vi "Load Config.vi"(8 "error in (no error)":errorcluster, 11 "SoftVar Module in":refnum<class "SoftVar Module.lvclass">) -> (0 "error out":errorcluster, 3 "SoftVar Module out":refnum<class "SoftVar Module.lvclass">)   [LabVIEW 2020, in "Volatus.lvlib" / "SoftVar Module.lvclass"]
uses:
  SoftVar Module.lvclass
  C:/dev/lv20CE/relink/lv-volatus/Volatus/Module/Module.lvclass
  Module/Module.lvclass/Module.ctl
  VolatusConfig/VolatusConfigElement/VolatusConfigElement.lvclass/VolatusConfigElement.ctl
  SoftVar Module.lvclass/SoftVar Module.ctl
  lv-vecto/Vecto/Group/Group.lvclass
  C:/dev/lv20CE/relink/lv-vecto/Vecto/GroupAbstract/GroupAbstract.lvclass
  Module/Config.vi
  VolatusConfig/VolatusConfigElement/Element.vi
  VolatusConfig/Task/Task.lvclass
  C:/dev/lv20CE/relink/lv-volatus/VolatusConfig/VolatusConfigElement/VolatusConfigElement.lvclass
  Module/Module.lvclass
  VolatusConfig/VolatusConfigElement/VolatusConfigElement.lvclass
  lv-cdm/CDM-Config/Config Element/Config Element.lvclass
  C:/dev/lv20CE/relink/lv-volatus/Volatus/SoftVar Module/SoftVar Module.lvclass
  VolatusConfig/Group/Group.lvclass
  VolatusConfig/Endpoint.ctl
  VolatusConfig/VolatusConfig.lvlib
  C:/dev/lv20CE/relink/lv-volatus/VolatusConfig/Task/Task.lvclass
  C:/dev/lv20CE/relink/lv-vecto/Vecto/Group/Group.lvclass
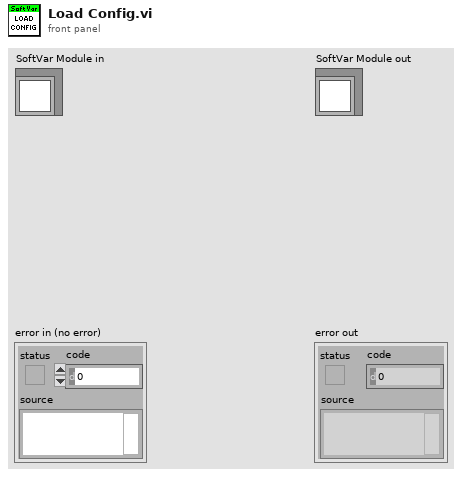
[diagram p1: front panel]
types:
  T1 = typedef "VolatusConfig.lvlib/Endpoint.ctl" = cluster{"Address":string, "Port":u16}
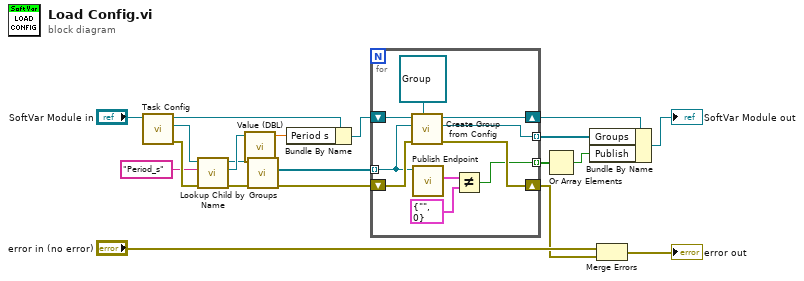
[diagram p0: block diagram]
diagram:
  n1 = call "Task Config.vi"("Module in"="SoftVar Module in") -> ("error out"=w20:errorcluster, "Task Config"=w16:refnum<class "Task.lvclass">, "Module out"=w17:refnum<class "SoftVar Module.lvclass">)  [unwired: 8 in]
  n2 = call "Lookup Child by Name.vi"("error in (no error)"=w20, "Child Name"="Period_s", "VolatusConfigElement in"=w16) -> ("error out"=w11:errorcluster, "Child"=w14:refnum<class "Config Element.lvclass">, "VolatusConfigElement out"=w12:refnum<class "Task.lvclass">)  [unwired: 5 in, 1 out]
  n3 = call "Value (DBL).vi"("Config Element in"=w14) -> ("DBL Value"=w13:dbl)  [unwired: 9 in, 1 out]
  n4 = call "Groups.vi"("error in (no error)"=w11, "Task in"=w12) -> ("error out"=w7:errorcluster, "Groups"=w8:refnum<class "Group.lvclass">[])  [unwired: 7 in, 1 out]
  n5 = Bundle By Name(cluster=w17, "Period s"=w13) -> (w10:refnum<class "SoftVar Module.lvclass">)
  n6 = for {
    shift-right: [w26] -> w9
    shift-left: w10 -> [w30]
    tunnel: w8 -> [w24] mode=indexing
    shift-right: [w27] -> w3
    shift-left: w7 -> [w28]
    tunnel: [w25] -> w5 mode=indexing
    tunnel: [w21] -> w2 mode=indexing
    n7 = call "Create Group from Config.vi"("Group Type (Abstract)"=refnum<class "Group.lvclass"> refnum ("Vecto.lvlib:Group.lvclass"), "error in (no error)"=w28, "Group Config"=w24, "Module in"=w30) -> ("error out"=w27:errorcluster, "Group"=w25:refnum<class "Group.lvclass">, "Module out"=w26:refnum<class "SoftVar Module.lvclass">)  [unwired: 5 in]
    n8 = call "Publish Endpoint.vi"("Group in"=w24) -> ("Publish Endpoint"=w23:T1)  [unwired: 8 in, 2 out]
    n9 = Not Equal?(x=w23, y=T1 {"Address"="", "Port"=0}) -> (x != y?=w21:bool)
  }
  n10 = Or Array Elements(Boolean array=w2) -> (logical OR=w1:bool)
  n11 = Bundle By Name(cluster=w9, "Groups"=w5, "Publish"=w1) -> (→"SoftVar Module out":refnum<class "SoftVar Module.lvclass">)
  n12 = Merge Errors("error in (no error)", w3) -> (→"error out":errorcluster)
